vi "dll_calc.vi"(8 "b":i32, 11 "a":i32) -> (0 "Division":sgl, 1 "Multiplication":i32, 2 "Subtract":i32, 3 "Sum":i32)   [LabVIEW 2021]
uses:
  <userlib>/new_libmath/new_libmath.lvlib
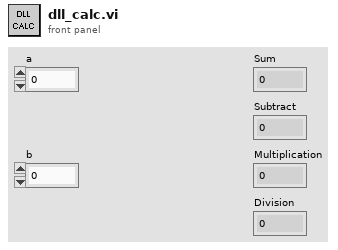
[diagram p1: front panel]
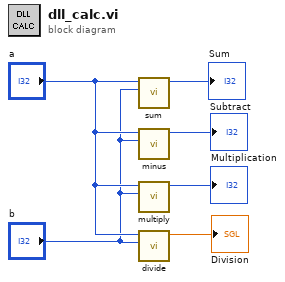
[diagram p0: block diagram]
diagram:
  n1 = call <userlib>:"sum.vi"("b"="b", "a"="a") -> ("function return"=→"Sum":i32)  [unwired: 8 in, 1 out]
  n2 = call <userlib>:"minus.vi"("b"="b", "a"="a") -> ("function return"=→"Subtract":i32)  [unwired: 8 in, 1 out]
  n3 = call <userlib>:"multiply.vi"("b"="b", "a"="a") -> ("function return"=→"Multiplication":i32)  [unwired: 8 in, 1 out]
  n4 = call <userlib>:"divide.vi"("b"="b", "a"="a") -> ("function return"=→"Division":sgl)  [unwired: 8 in, 1 out]
